vi "GitServer_MAIN.vi"() -> ()   [LabVIEW 2018]
panel:
  out "Add":dbl
  in  "Numeric 2":dbl
  in  "Numeric 1":dbl
  out "i":i32
  in  "stop":bool
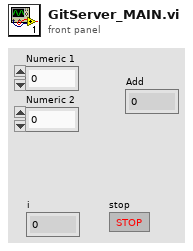
[diagram p1: front panel]
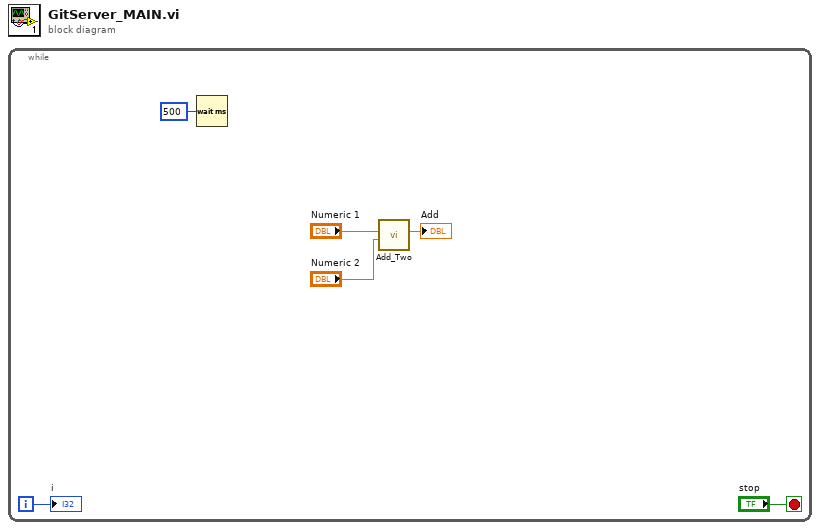
[diagram p0: block diagram]
diagram:
  n1 = while {
    i -> [w5]
    stop <- "stop" stop-if-true
    n2 = Wait (ms)(milliseconds to wait=u32 500) -> ()  [unwired: 1 out]
    n3 = call "Add_Two.vi"("Numeric 2"="Numeric 2", "Numeric 1"="Numeric 1") -> ("Add"=→"Add":dbl)  [unwired: 9 in]
    "i" <- w5
  }
